vi "exp1.vi"() -> ()   [LabVIEW 2014]
panel:
  in  "采集的电压":dbl
  out "温度值":dbl
  in  "温度值单位":bool
  out "温度计":dbl(slide) scale=0.0..100.0
  # "摄氏"
  # "华氏"
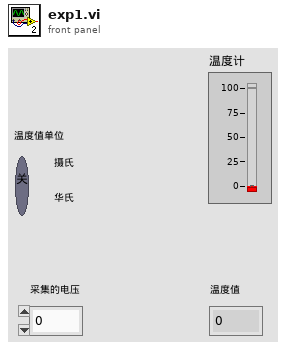
[diagram p1: front panel]
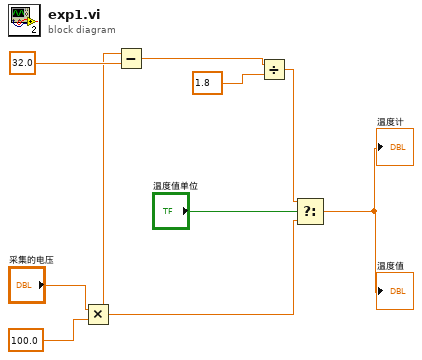
[diagram p0: block diagram]
diagram:
  n1 = Multiply(x="采集的电压", y=100.0) -> (x*y=w3:dbl)
  n2 = Subtract(x=w3, y=32.0) -> (x-y=w6:dbl)
  n3 = Divide(x=w6, y=1.8) -> (x/y=w2:dbl)
  n4 = Select(t=w2, s="温度值单位", f=w3) -> (s? t:f=→"温度计" →"温度值":dbl)
